vi "Main.vi"(8 "error in (no error)":errorcluster, 11 "Event Registration Refnum":refnum<event-registration>) -> (0 "error out":errorcluster)   [LabVIEW 2023, in "Template.lvlib"]
uses:
  Template.lvlib
  Type Def/Module Data.ctl
panel:
  in  "stop":bool
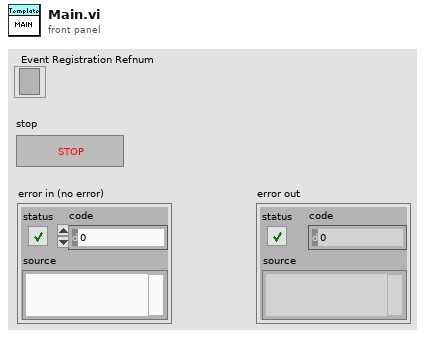
[diagram p1: front panel]
types:
  T1 = typedef "Template.lvlib/Module Data.ctl" = cluster{"Module Name":string}
  T2 = typedef "Template.lvlib/Message Data.ctl" = cluster{"Message":string, "Data":variant}
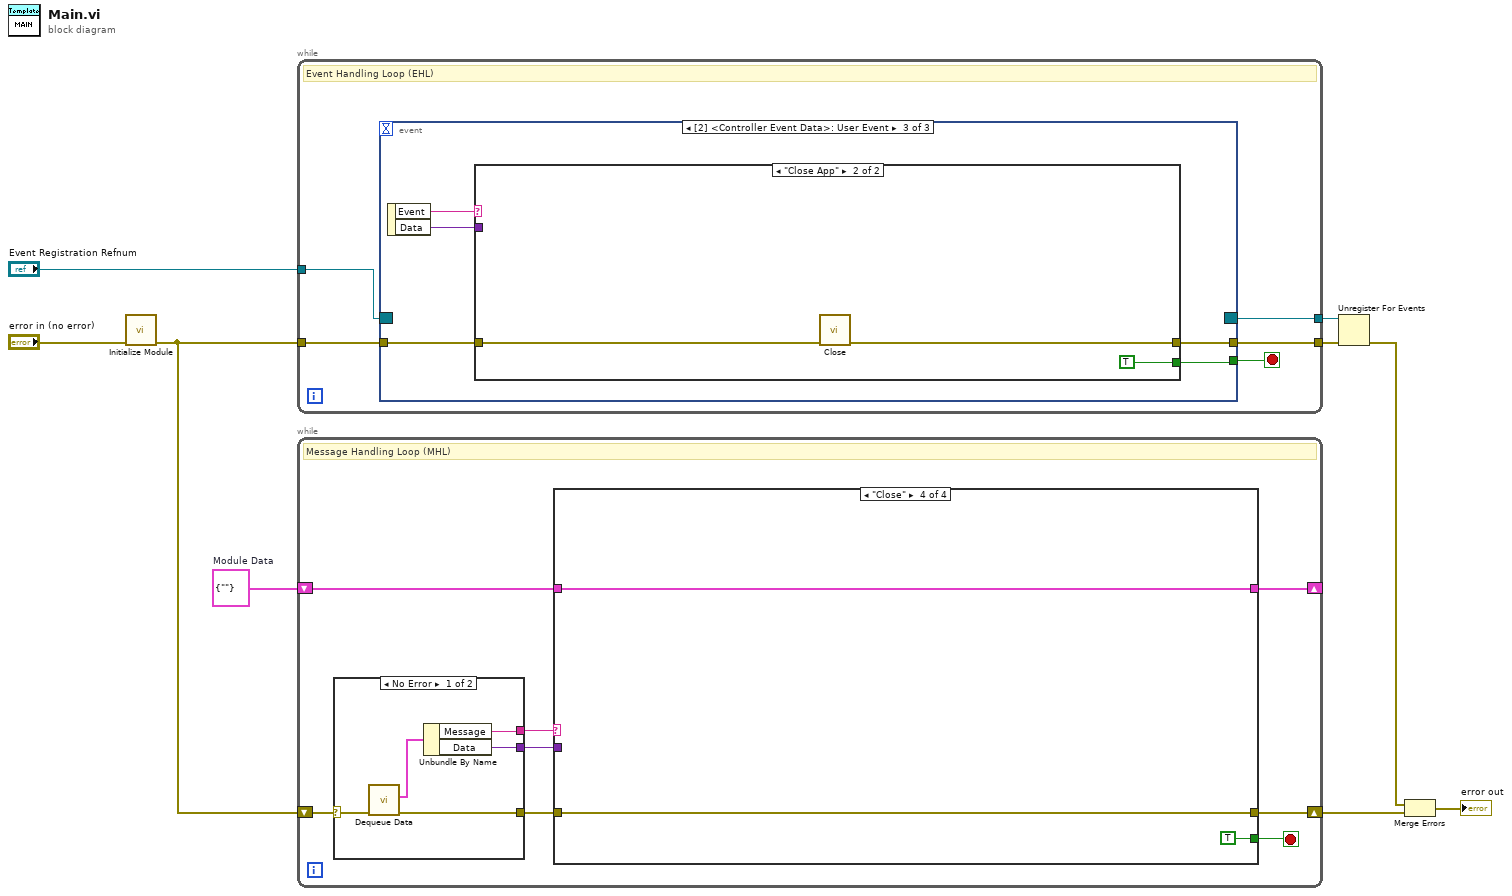
[diagram p0: block diagram]
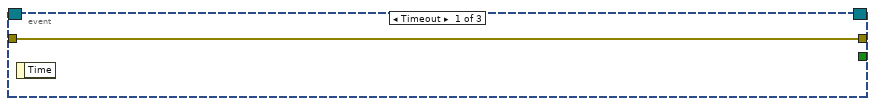
[diagram p2: hidden frame]
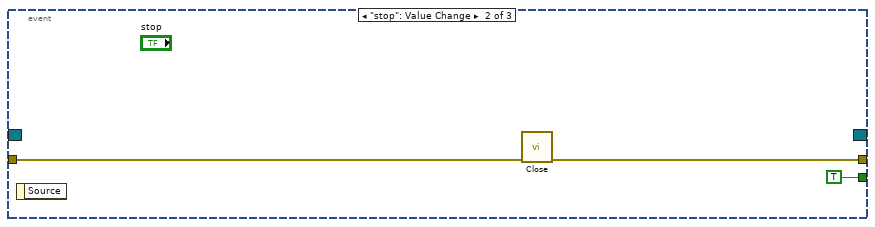
[diagram p3: hidden frame]
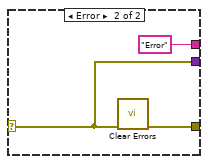
[diagram p5: hidden frame]
diagram:
  w8 = T1 {"Module Name"=""}  # Module Data
  n1 = call "Initialize Module.vi"("error in (no error)"="error in (no error)") -> ("error out"=w7:errorcluster)  [unwired: 10 in]
  n2 = while {
    tunnel: w7 -> [w14]
    tunnel: [w13] -> w4
    tunnel: [w12] -> w2
    tunnel: "Event Registration Refnum" -> [w10]
    stop <- w11 stop-if-true
    # "Event Handling Loop (EHL)"
    n3 = event shown="[2] <Controller Event Data>: User Event" {
      selector: w10 -> [_ _ _]
      dyn-events: [_ _ _] -> w12
      timeout: _ -> [_ _ _]
      tunnel: w14 -> [w15 w18 w21]
      tunnel: [w15 w17 w20] -> w13
      tunnel: [_ TRUE w19] -> w11
      event Timeout {
        n4 = event-data() -> ()  [unwired: 1 in, 1 out]
      }
      event "stop": Value Change {
        n5 = event-data() -> ()  [unwired: 1 in, 1 out]
        n6 = call "Close.vi"("error in (no error)"=w18) -> ("error out"=w17:errorcluster)  [unwired: 10 in]
      }
      event User Event {
        n7 = event-data() -> ("Event"=w23:string, "Data"=w22:variant)  [unwired: 1 in]
        n8 = case shown="\"Close App\"" w23 {
          tunnel: w22 -> [_ _]
          tunnel: w21 -> [w24 w26]
          tunnel: [w24 w25] -> w20
          tunnel: [_ TRUE] -> w19
          frame "False", Default {
          }
          frame "Close App" {
            n9 = call "Close.vi"("error in (no error)"=w26) -> ("error out"=w25:errorcluster)  [unwired: 10 in]
          }
        }
      }
    }
  }
  n10 = while {
    shift-right: [w34] -> _
    shift-left: w8 -> [w35]
    shift-right: [w29] -> w6
    shift-left: w7 -> [w33]
    stop <- w28 stop-if-true
    # "Message Handling Loop (MHL)"
    n11 = case shown="No Error" w33 {
      selector: w33 -> [w40 w41]
      tunnel: [w38 "Error" ("Message")] -> w32
      tunnel: [w37 w41] -> w31
      tunnel: [w36 w42] -> w30
      frame No Error {
        n12 = call "Dequeue Data.vi"("error in (no error)"=w40) -> ("error out"=w36:errorcluster, "Message Data"=w39:T2)  [unwired: 9 in]
        n13 = Unbundle By Name(w39) -> ("Message"=w38:string, "Data"=w37:variant)
      }
      frame Error {
        n14 = call <vilib>:"Clear Errors.vi"("error in (no error)"=w41) -> ("error out"=w42:errorcluster)  [unwired: 5 in, 1 out]
      }
    }
    n15 = case shown="\"Close\"" w32 {
      tunnel: w35 -> [w45 w47 w49 w52]
      tunnel: [w45 w47 w49 w52] -> w34
      tunnel: w31 -> [_ _ _ _]
      tunnel: w30 -> [w44 w46 w48 w51]
      tunnel: [w44 w46 w48 w51] -> w29
      tunnel: [_ _ _ TRUE] -> w28
      frame "False", Default {
      }
      frame "Init" {
      }
      frame "Error" {
      }
      frame "Close" {
      }
    }
  }
  n16 = Unregister For Events(event registration refnum=w2, error in=w4) -> (error out=w3:errorcluster)
  n17 = Merge Errors(w3, w6) -> (→"error out":errorcluster)
